vi "Main Tclk.vi"() -> ()   [LabVIEW 2018] (continued)
            n4776 = event-data() -> ()  [unwired: 5 out]
            n4777 = local read "SEM Scan Parameters"() -> (w3782:T26)
            n4778 = Unbundle By Name(w3782) -> ("X stig"=w3784:sgl[][], "X tiles"=w3780:u8, "Y tiles"=w3779:u8)
            n4779 = call "2D array edit.vi"("Data Entry Limits:Increment"=0.1, "Display Format:Precision"=u8 2, "Rows"=w3779, "Columns"=w3780, "Caption.Text"="X stig (%)", "Input array"=w3784) -> ("Output array"=w3777:sgl[][])  [unwired: 5 in]
            n4780 = Array Size(array=w3777) -> (size(s)=w3778:i32[])
            n4781 = Index Array(array=w3778) -> (element #1=w3776:i32, element #2=w3775:i32)  [unwired: 2 in]
            n4782 = Bundle By Name(cluster=w3782, "X stig"=w3777, "X tiles"=w3775, "Y tiles"=w3776) -> (w3781:T26)
            n4783 = local write "SEM Scan Parameters"(w3781) -> ()
          }
          event "SEM Scan Parameters.Y stig": Mouse Down; "SEM Scan Parameters.Y stig": Value Change {
            n4784 = event-data() -> ()  [unwired: 5 out]
            n4785 = local read "SEM Scan Parameters"() -> (w3794:T26)
            n4786 = Unbundle By Name(w3794) -> ("Y stig"=w3796:sgl[][], "X tiles"=w3792:u8, "Y tiles"=w3791:u8)
            n4787 = call "2D array edit.vi"("Data Entry Limits:Increment"=0.1, "Display Format:Precision"=u8 2, "Rows"=w3791, "Columns"=w3792, "Caption.Text"="Y stig (%)", "Input array"=w3796) -> ("Output array"=w3789:sgl[][])  [unwired: 5 in]
            n4788 = Array Size(array=w3789) -> (size(s)=w3790:i32[])
            n4789 = Index Array(array=w3790) -> (element #1=w3788:i32, element #2=w3787:i32)  [unwired: 2 in]
            n4790 = Bundle By Name(cluster=w3794, "Y stig"=w3789, "X tiles"=w3787, "Y tiles"=w3788) -> (w3793:T26)
            n4791 = local write "SEM Scan Parameters"(w3793) -> ()
          }
          event "SEM Scan Parameters.X aln": Mouse Down; "SEM Scan Parameters.X aln": Value Change {
            n4792 = event-data() -> ()  [unwired: 5 out]
            n4793 = local read "SEM Scan Parameters"() -> (w3806:T26)
            n4794 = Unbundle By Name(w3806) -> ("X aln"=w3808:sgl[][], "X tiles"=w3804:u8, "Y tiles"=w3803:u8)
            n4795 = call "2D array edit.vi"("Data Entry Limits:Increment"=0.1, "Display Format:Precision"=u8 2, "Rows"=w3803, "Columns"=w3804, "Caption.Text"="X aln (%)", "Input array"=w3808) -> ("Output array"=w3801:sgl[][])  [unwired: 5 in]
            n4796 = Array Size(array=w3801) -> (size(s)=w3802:i32[])
            n4797 = Index Array(array=w3802) -> (element #1=w3800:i32, element #2=w3799:i32)  [unwired: 2 in]
            n4798 = Bundle By Name(cluster=w3806, "X aln"=w3801, "X tiles"=w3799, "Y tiles"=w3800) -> (w3805:T26)
            n4799 = local write "SEM Scan Parameters"(w3805) -> ()
          }
          event "SEM Scan Parameters.Y aln": Mouse Down; "SEM Scan Parameters.Y aln": Value Change {
            n4800 = event-data() -> ()  [unwired: 5 out]
            n4801 = local read "SEM Scan Parameters"() -> (w3818:T26)
            n4802 = Unbundle By Name(w3818) -> ("Y aln"=w3820:sgl[][], "X tiles"=w3816:u8, "Y tiles"=w3815:u8)
            n4803 = call "2D array edit.vi"("Data Entry Limits:Increment"=0.1, "Display Format:Precision"=u8 2, "Rows"=w3815, "Columns"=w3816, "Caption.Text"="Y aln (%)", "Input array"=w3820) -> ("Output array"=w3813:sgl[][])  [unwired: 5 in]
            n4804 = Array Size(array=w3813) -> (size(s)=w3814:i32[])
            n4805 = Index Array(array=w3814) -> (element #1=w3811:i32, element #2=w3812:i32)  [unwired: 2 in]
            n4806 = Bundle By Name(cluster=w3818, "Y aln"=w3813, "X tiles"=w3812, "Y tiles"=w3811) -> (w3817:T26)
            n4807 = local write "SEM Scan Parameters"(w3817) -> ()
          }
          event "SEM Scan Parameters.dX (um)": Mouse Down {
            w3823 = u8 1 ("Rows")
            n4808 = event-data() -> ()  [unwired: 9 out]
            n4809 = local read "SEM Scan Parameters"() -> (w3831:T26)
            n4810 = local write "Delta X array for stop limit"(sgl[] [] ("Delta X array for stop limit")) -> ()
            n4811 = Unbundle By Name(w3831) -> ("dX (um)"=w3827:sgl[], "Y tiles"=w3822:u8)
            n4812 = Reshape Array(w3827, w3822, w3823) -> (w3826:sgl[][])
            n4813 = call "2D array edit.vi"("Data Entry Limits:Increment"=0.1, "Display Format:Precision"=u8 2, "Rows"=w3822, "Columns"=w3823, "Caption.Text"="dX (um)", "Input array"=w3826) -> ("Output array"=w3825:sgl[][])  [unwired: 5 in]
            n4814 = Reshape Array(w3825, w3822) -> (w3824:sgl[])
            n4815 = Bundle By Name(cluster=w3831, "dX (um)"=w3824, "Y tiles"=w3822) -> (w3830:T26)
            n4816 = local write "SEM Scan Parameters"(w3830) -> ()
          }
          event "SEM Scan Parameters.dY (um)": Mouse Down {
            w3838 = u8 1 ("Rows")
            n4817 = event-data() -> ()  [unwired: 9 out]
            n4818 = local read "SEM Scan Parameters"() -> (w3843:T26)
            n4819 = local write "Delta Y array for stop limit"(sgl[] [] ("Delta X array for stop limit")) -> ()
            n4820 = Unbundle By Name(w3843) -> ("dY (um)"=w3839:sgl[], "X tiles"=w3834:u8)
            n4821 = Reshape Array(w3839, w3838, w3834) -> (w3837:sgl[][])
            n4822 = call "2D array edit.vi"("Data Entry Limits:Increment"=0.1, "Display Format:Precision"=u8 2, "Rows"=w3838, "Columns"=w3834, "Caption.Text"="dY (um)", "Input array"=w3837) -> ("Output array"=w3836:sgl[][])  [unwired: 5 in]
            n4823 = Reshape Array(w3836, w3834) -> (w3835:sgl[])
            n4824 = Bundle By Name(cluster=w3843, "dY (um)"=w3835, "X tiles"=w3834) -> (w3842:T26)
            n4825 = local write "SEM Scan Parameters"(w3842) -> ()
          }
          event "X shift (nm/image)": Mouse Down {
            n4826 = event-data() -> ()  [unwired: 9 out]
            n4827 = local read "X shift (nm/image)"() -> (w3848:sgl)
            n4828 = local read "Remaining X shift frames"() -> (w3845:u32)
            n4829 = Compound Arithmetic op=MULTIPLY(w3848, sgl 0.001 ("value"), w3845) -> (w3849:sgl)
            n4830 = call "Image shift dialog.vi"("Remaining shift (um)"=w3849, "Image shift"=w3848, "Caption.Text"="X shift (nm/image)") -> ("Image shift (nm/image)"=w3850:sgl, "Remaining shift frames"=w3847:u32)  [unwired: 7 in]
            n4831 = local write "Remaining X shift frames"(w3847) -> ()
            n4832 = local write "X shift (nm/image)"(w3850) -> ()
          }
          event "Y shift (nm/image)": Mouse Down; "Y shift (nm/image)": Value Change {
            n4833 = event-data() -> ()  [unwired: 5 out]
            n4834 = local read "Y shift (nm/image)"() -> (w3855:sgl)
            n4835 = local read "Remaining Y shift frames"() -> (w3854:u32)
            n4836 = Compound Arithmetic op=MULTIPLY(w3855, sgl 0.001 ("value"), w3854) -> (w3856:sgl)
            n4837 = call "Image shift dialog.vi"("Remaining shift (um)"=w3856, "Image shift"=w3855, "Caption.Text"="Y shift (nm/image)") -> ("Image shift (nm/image)"=w3858:sgl, "Remaining shift frames"=w3853:u32)  [unwired: 7 in]
            n4838 = local write "Remaining Y shift frames"(w3853) -> ()
            n4839 = local write "Y shift (nm/image)"(w3858) -> ()
          }
          event "Mill": Value Change {
            n4840 = event-data() -> ("NewVal"=w3859:bool)  [unwired: 6 out]
            n4841 = case shown="True" w3859 {
              frame False {
                n4842 = local read "Original WatchDog Mode"() -> (w3860:u16)
                n4843 = shared-variable "My Computer\\Zeiss Library.lvlib\\Milling Stop"(TRUE ("Milling Stop")) -> ()  [unwired: 1 in, 1 out]
                n4844 = local write "WatchDog Mode"(w3860) -> ()
              }
              frame True {
                n4845 = stacked-sequence {
                  frame #0 {
                    n4846 = local read "WatchDog Mode"() -> (→"Original WatchDog Mode":u16)
                  }
                  frame #1 {
                    w3863 = u16 0 items=["Do Nothing", "Send Idle Only", "Watch FIB & SEM", "Watch FIB Only", "Watch SEM Only"] ("WatchDog Mode")
                    n4847 = local write "WatchDog Mode"(w3863) -> ()
                  }
                }
              }
            }
          }
          event "Mill Manual Pause": Value Change {
            w3869 = u8 0 ("AF Count")
            w3871 = FALSE ("Reset WD")
            w3870 = TRUE ("Reset WD")
            n4848 = event-data() -> ("NewVal"=w3872:bool)  [unwired: 5 out]
            n4849 = case shown="False" w3872 {
              frame False {
                n4850 = local read "Status message"() -> (w3883:string)
                n4851 = local read "Last milling snapshot"() -> (w3876:path)
                n4852 = Equal?(x=w3883, y="Manual pausing ..." ("Status message")) -> (x = y?=w3882:bool)
                n4853 = call-poly <vilib>:"Read From XML File.vi"("XML File Path"=w3876) -> ("XML Elements"=w3875:string)  [unwired: 8 in, 2 out]
                n4854 = Unflatten From XML(xml string=w3875, type=T46 {"Timestamp"=timestamp(0 s since 1904-01-01), "Milling Z voltage"=0.0, "FIB slice #"=0, "Pause for reheat"=FALSE, "Last good FI"=0.0, "Focus index"=0.0, "SEM max FOV"=0.0, "Remaining X shift frames"=0, "Remaining Y shift frames"=0} ("output cluster")) -> (value=w3877:T46)  [unwired: 1 in, 1 out]
                n4855 = Select(t="SEM between FIB" ("Status message"), s=w3882, f="Resume FIB milling ..." ("Status message")) -> (s? t:f=w3881:string)
                n4856 = Unbundle By Name(w3877) -> ("Milling Z voltage"=w3873:sgl)
                n4857 = shared-variable ".\\Zeiss Library.lvlib\\Milling Z Voltage Last"(w3873) -> ()  [unwired: 1 in, 1 out]
                n4858 = local write "Status message"(w3881) -> ()
              }
              frame True {
                n4859 = local read "Status message"() -> (w3889:string)
                n4860 = Equal?(x=w3889, y="SEM between FIB" ("Status message")) -> (x = y?=w3886:bool)
                n4861 = Select(t="Manual pausing ..." ("Status message"), s=w3886, f="Manual paused" ("Status message")) -> (s? t:f=w3885:string)
                n4862 = local write "Status message"(w3885) -> ()
              }
            }
            n4863 = local write "SW error warning armed"(w3870) -> ()
            n4864 = local write "Auto Focus"(w3871) -> ()
            n4865 = local write "Auto Stig"(w3871) -> ()
            n4866 = local write "Auto Align"(w3871) -> ()
            n4867 = local write "Reset Focus"(w3870) -> ()
            n4868 = local write "3D image paused armed"(w3870) -> ()
            n4869 = local write "Temperature warning armed"(w3870) -> ()
            n4870 = local write "AF Count"(w3869) -> ()
            n4871 = local write "AS Count"(w3869) -> ()
            n4872 = local write "AA Count"(w3869) -> ()
            n4873 = local read "SEM Scan Parameters"() -> (w3865:T26)
            n4874 = Unbundle By Name(w3865) -> ("Y tiles"=w3866:u8, "X tiles"=w3867:u8)
            n4875 = Initialize Array(FALSE ("ASX Success"), w3866, w3867) -> (w3868:bool[][])
            n4876 = local write "AAY Success tiled"(w3868) -> ()
            n4877 = local write "AF Success tiled"(w3868) -> ()
            n4878 = local write "ASX Success tiled"(w3868) -> ()
            n4879 = local write "ASY Success tiled"(w3868) -> ()
            n4880 = local write "AAX Success tiled"(w3868) -> ()
          }
          event "Mill Stop": Value Change {
            n4881 = event-data() -> ("NewVal"=w3890:bool)  [unwired: 6 out]
            n4882 = case shown="True" w3890 {
              frame False {
              }
              frame True {
                n4883 = local read "Original WatchDog Mode"() -> (w3891:u16)
                n4884 = shared-variable "My Computer\\Zeiss Library.lvlib\\Milling Stop"(TRUE ("Milling Stop")) -> ()  [unwired: 1 in, 1 out]
                n4885 = local write "WatchDog Mode"(w3891) -> ()
              }
            }
          }
          event "Save Probe Table": Value Change {
            n4886 = event-data() -> ("NewVal"=w3893:bool)  [unwired: 5 out]
            n4887 = case shown="True" w3893 {
              frame False {
              }
              frame True {
                n4888 = Two Button Dialog(message="Save FIB Probe Table?") -> (T button?=w3894:bool)  [unwired: 2 in]
                n4889 = case shown="True" w3894 {
                  frame False {
                    n4890 = local write "Save Probe Table"(FALSE ("Min FIB probe")) -> ()
                  }
                  frame True {
                    n4891 = stacked-sequence {
                      frame #0 {
                        n4892 = local read "Api"() -> (w3898:refnum<k7>)
                        n4893 = local read "FIB Milling Probe"() -> (w3897:string)
                        n4894 = call "SmartSEM Remote API save FIB probe table.vi"("FIB Probe"=w3897, "ActiveX Container"=w3898) -> ()  [unwired: 8 in, 2 out]
                        n4895 = local write "Status message"("Measuring FIB probe currents" ("Status message")) -> ()
                      }
                      frame #1 {
                        n4896 = local write "Save Probe Table"(FALSE ("Min FIB probe")) -> ()
                        n4897 = local write "Status message"("FIB Probe Table saved" ("Status message")) -> ()
                      }
                    }
                  }
                }
              }
            }
          }
          event "FIB Milling Probe": Value Change {
            n4898 = event-data() -> ()  [unwired: 6 out]
            n4899 = local read "Machine Type"() -> (w3902:u8)
            n4900 = case shown="2" w3902 {
              frame 0, Default {
              }
              frame 2 {
                n4901 = local read "Api"() -> (w3909:refnum<k7>)
                n4902 = call "SmartSEM Remote API set string.vi"("vValue"="FIB Milling Probe", "lpszParam"="DP_FIB_IMAGE_PROBE", "ActiveX Container"=w3909) -> ("error out"=w3903:errorcluster, "reference out"=w3906:refnum<k7>)  [unwired: 7 in]
                n4903 = call "SmartSEM Remote API set string.vi"("error in"=w3903, "vValue"="Undefined", "lpszParam"="DP_FIB_MILL_PROBE", "ActiveX Container"=w3906) -> ()  [unwired: 6 in, 2 out]
              }
            }
          }
          event "Min FIB probe": Value Change {
            n4904 = event-data() -> ("NewVal"=w3910:bool)  [unwired: 5 out]
            n4905 = case shown="True" w3910 {
              frame False {
              }
              frame True {
                n4906 = Two Button Dialog(message="Switch to min current of the same probe size?") -> (T button?=w3911:bool)  [unwired: 2 in]
                n4907 = case shown="True" w3911 {
                  frame False {
                    n4908 = local write "Min FIB probe"(FALSE ("Min FIB probe")) -> ()
                  }
                  frame True {
                    n4909 = stacked-sequence {
                      frame #0 {
                        n4910 = local read "Api"() -> (w3916:refnum<k7>)
                        n4911 = local read "FIB Milling Probe"() -> (w3917:string)
                        n4912 = local write "Min FIB probe"(FALSE ("Min FIB probe")) -> ()
                        n4913 = call "SmartSEM Remote API goto min or max FIB probe current.vi"("Min or Max"="Min", "FIB Probe"=w3917, "ActiveX Container"=w3916) -> ("Goto probe"=w3914:string)  [unwired: 7 in, 1 out]
                        n4914 = local write "FIB Milling Probe"(w3914) -> ()
                        n4915 = local write "Status message"("Measuring FIB probe currents" ("Status message")) -> ()
                      }
                      frame #1 {
                        n4916 = local write "Status message"("Switched to minimal current of the same probe" ("Status message")) -> ()
                      }
                    }
                  }
                }
              }
            }
          }
          event "Max FIB probe": Value Change {
            n4917 = event-data() -> ("NewVal"=w3921:bool)  [unwired: 5 out]
            n4918 = case shown="True" w3921 {
              frame False {
              }
              frame True {
                n4919 = Two Button Dialog(message="Switch to max current of the same probe size?") -> (T button?=w3922:bool)  [unwired: 2 in]
                n4920 = case shown="True" w3922 {
                  frame False {
                    n4921 = local write "Max FIB probe"(FALSE ("Min FIB probe")) -> ()
                  }
                  frame True {
                    n4922 = stacked-sequence {
                      frame #0 {
                        n4923 = local read "Api"() -> (w3928:refnum<k7>)
                        n4924 = local read "FIB Milling Probe"() -> (w3927:string)
                        n4925 = local write "Max FIB probe"(FALSE ("Min FIB probe")) -> ()
                        n4926 = call "SmartSEM Remote API goto min or max FIB probe current.vi"("Min or Max"="Max", "FIB Probe"=w3927, "ActiveX Container"=w3928) -> ("Goto probe"=w3926:string)  [unwired: 7 in, 1 out]
                        n4927 = local write "FIB Milling Probe"(w3926) -> ()
                        n4928 = local write "Status message"("Measuring FIB probe currents" ("Status message")) -> ()
                      }
                      frame #1 {
                        n4929 = local write "Status message"("Switched to maximal current of the same probe" ("Status message")) -> ()
                      }
                    }
                  }
                }
              }
            }
          }
          event "FIB time lapse": Value Change {
            n4930 = event-data() -> ("NewVal"=w3932:bool)  [unwired: 5 out]
            n4931 = case shown="False" w3932 {
              frame False {
                n4932 = stacked-sequence {
                  frame #0 {
                    n4933 = local read "FIB HW Config"() -> (w3935:T23)
                    n4934 = Unbundle By Name(w3935) -> ("Beam blank"=w3936:tag)
                    n4935 = local read "Api"() -> (w3933:refnum<k7>)
                    n4936 = call "FIB beam blank.vi"("ActiveX Container"=w3933, "Beam blanked"=TRUE ("Ext on"), "lines"=w3936) -> ()  [unwired: 2 in, 1 out]
                  }
                  frame #1 {
                    n4937 = local read "SEM HW Config"() -> (w3941:T9)
                    n4938 = Unbundle By Name(w3941) -> ("Detector FIB-NI auto switch"=w3942:tag)
                    n4939 = call-poly <vilib>:"DAQmx Create Virtual Channel.vi"("lines"=w3942) -> ("task out"=w3939:refnum<k21>, "error out"=w3940:errorcluster)  [unwired: 4 in, 9 out]
                    n4940 = call-poly <vilib>:"DAQmx Write.vi"("task/channels in"=w3939, "data"=FALSE, "error in"=w3940) -> ("task out"=w3937:refnum<k21>, "error out"=w3938:errorcluster)  [unwired: 1 in, 10 out]
                    n4941 = call <vilib>:"DAQmx Clear Task.vi"("task in"=w3937, "error in"=w3938) -> ()  [unwired: 14 out]
                  }
                  frame #2 {
                    n4942 = local read "FIB HW Config"() -> (w3946:T23)
                    n4943 = Unbundle By Name(w3946) -> ("FIB Ext Scan"=w3945:tag)
                    n4944 = call "FIB ext scan.vi"("Ext on"=FALSE, "FIB Ext Scan"=w3945) -> ()  [unwired: 9 in, 1 out]
                  }
                  frame #3 {
                    n4945 = local read "Machine Type"() -> (w3947:u8)
                    n4946 = case shown="2" w3947 {
                      frame 0, Default {
                      }
                      frame 1 {
                        w3948 = TRUE ("Initialization")
                        n4947 = local read "COM port"() -> (w3954:refnum<visa-resource-name>)
                        n4948 = call "FIB mode.vi"("Initialization"=w3948, "FIB mode"=T10."SEM", "COM port in"=w3954) -> ("COM port out"=w3953:refnum<visa-resource-name>)  [unwired: 7 in, 1 out]
                        n4949 = call "Remcon32 command.vi"("SEM command"="edx 0", "COM port in"=w3953) -> ("COM port out"=w3952:refnum<visa-resource-name>)  [unwired: 6 in, 3 out]
                        n4950 = call "Remcon32 command.vi"("Close session"=w3948, "SEM command"="frez", "COM port in"=w3952) -> ()  [unwired: 5 in, 4 out]
                      }
                      frame 2 {
                        n4951 = local read "Api"() -> (w3955:refnum<k7>)
                        n4952 = call "SmartSEM Remote API set float.vi"("vValue"=sgl 2.0, "lpszParam"="DP_FIB_BLANKER_MODE" ("lpszCommand"), "ActiveX Container"=w3955) -> ("error out"=w3956:errorcluster, "reference out"=w3957:refnum<k7>)  [unwired: 7 in]
                        n4953 = call "SmartSEM Remote API FIB mode.vi"("error in"=w3956, "FIB mode"=T50."SEM", "ActiveX Container"=w3957) -> ("error out"=w3960:errorcluster, "reference out"=w3961:refnum<k7>)  [unwired: 7 in]
                        n4954 = invoke class="_EMApi" method="Execute"(reference=w3961, error in=w3960, "lpszCommand"="CMD_FREEZE_ALL") -> ()  [unwired: 1 in, 4 out]
                      }
                    }
                  }
                  frame #4 {
                    n4955 = local write "Status message"("standby" ("Status message")) -> ()
                  }
                }
              }
              frame True {
              }
            }
          }
          event "FIB Image": Mouse Down {
            n4956 = event-data() -> ("Coords"=→"Mouse Down Coords":T22)  [unwired: 3 out]
            n4957 = register-events(reference=w3973, w3969) -> (reference out=w3972:refnum<event-registration>, error out=w3971:errorcluster)  [unwired: 1 in]
            n4958 = local read "Spot"() -> (w3968:bool)
            n4959 = property on="Cursor Z (V)" class="DigNum (strict)"("Visible"=FALSE) -> ()  [unwired: 2 in, 2 out]
            n4960 = case shown="False" w3968 {
              frame False {
              }
              frame True {
                n4961 = local read "FIB HW Config"() -> (w3977:T23)
                n4962 = Unbundle By Name(w3977) -> ("Beam blank"=w3976:tag)
                n4963 = local read "Api"() -> (w3974:refnum<k7>)
                n4964 = call "FIB beam blank.vi"("ActiveX Container"=w3974, "Beam blanked"=TRUE, "lines"=w3976) -> ()  [unwired: 2 in, 1 out]
              }
            }
            "Mouse down" <- TRUE ("Mouse down")
          }
          event "FIB Image": Mouse Move {
            n4965 = event-data() -> ("Coords"=w3982:T22)  [unwired: 1 out]
            n4966 = local read "Mouse down"() -> (w3981:bool)
            n4967 = local read "Spot"() -> (w3980:bool)
            n4968 = local read "FIB"() -> (w3979:bool)
            n4969 = Or(x=w3980, y=w3979) -> (x .or. y?=w3978:bool)
            n4970 = case shown="False" w3981 {
              tunnel: [w4009 w4013] -> w3984
              tunnel: w3983 -> [w4009 w4012]
              tunnel: w3982 -> [w4008 w4011]
              tunnel: w3978 -> [_ w4010]
              frame False {
                w3985 = i16 0 ("upper limit")
                n4971 = property on="FIB Image" class="IntGraph (strict)"() -> ("Plot Bounds"=w4007:T70, "Width"=w3989:u32, "Height"=w3997:u32)  [unwired: 2 in, 2 out]
                n4972 = local read "FIB Scan Parameters"() -> (w4006:T32)
                n4973 = Unbundle By Name(w4007) -> ("Right"=w3992:i16, "Bottom"=w4000:i16)
                n4974 = Unbundle By Name(w4008) -> ("Horizontal"=w3991:i32, "Vertical"=w3993:i32)
                n4975 = Unbundle By Name(w4006) -> ("Z size (V)"=w3999:dbl)
                n4976 = To Word Integer(number=w3997) -> (16bit integer=w3995:i16)
                n4977 = To Word Integer(number=w3993) -> (16bit integer=w3994:i16)
                n4978 = Subtract(x=w3992, y=w3991) -> (x-y=w3990:i32)
                n4979 = Subtract(x=w4000, y=w3994) -> (x-y=w3996:i16)
                n4980 = In Range and Coerce(upper limit=w3989, x=w3990, lower limit=w3985) -> (In Range?=w3988:bool)  [unwired: 1 out]
                n4981 = In Range and Coerce(upper limit=w3995, x=w3996, lower limit=w3985) -> (coerced(x)=w3998:i16, In Range?=w3987:bool)
                n4982 = Multiply(x=w3998, y=w3999) -> (x*y=w4005:dbl)
                n4983 = Multiply(x=w3999, y=0.5) -> (x*y=w4003:dbl)
                n4984 = And(x=w3988, y=w3987) -> (x .and. y?=w3986:bool)
                n4985 = Divide(x=w4005, y=w3997) -> (x/y=w4004:dbl)
                n4986 = property on="Cursor Z (V)" class="DigNum (strict)"("Visible"=w3986) -> ()  [unwired: 2 in, 2 out]
                n4987 = Subtract(x=w4004, y=w4003) -> (x-y=→"Cursor Z (V)":dbl)
              }
              frame True {
                n4988 = case shown="False" w4010 {
                  tunnel: w4011 -> [w4015 _]
                  tunnel: [w4014 w4138] -> w4013
                  tunnel: w4012 -> [_ w4138]
                  frame False {
                    n4989 = stacked-sequence {
                      tunnel: w4015 -> [_ w4020]
                      tunnel: [_ w4018] -> w4014
                      frame #0 {
                        n4990 = call <vilib>:"Draw Rectangle.vi"("picture"=picture data[5B]) -> ("new picture"=w4017:picture)  [unwired: 8 in]
                        n4991 = property on="FIB Image" class="IntGraph (strict)"("PlotImages.Front"=w4017) -> ()  [unwired: 2 in, 2 out]
                      }
                      frame #1 {
                        n4992 = case shown="True" "ROI" {
                          tunnel: w4020 -> [w4062 w4129]
                          tunnel: [w4021 w4073] -> w4018
                          frame False {
                            w4039 = 5 ("dimension size")
                            w4060 = u32 16711680 ("color(black)")
                            n4993 = local read "Mouse Down Coords"() -> (w4063:T22)
                            n4994 = Subtract(x=w4062, y=w4063) -> (x-y=w4061:T22)
                            n4995 = Unbundle By Name(w4061) -> ("Horizontal"=w4040:i32, "Vertical"=w4038:i32)
                            n4996 = Initialize Array(w4040, w4039) -> (w4037:i32[])
                            n4997 = Initialize Array(w4038, w4039) -> (w4036:i32[])
                            n4998 = local read "FIB Scan Parameters"() -> (w4050:T32)
                            n4999 = local read "Milling para"() -> (w4055:T35)
                            n5000 = local read "FIB Options"() -> (w4056:T33)
                            n5001 = local read "Trapezoidal"() -> (w4022:cluster{"X":i16, "Y":i16}[])
                            n5002 = Build Cluster Array(w4037, w4036) -> (w4035:cluster{"Horizontal":i32, "Vertical":i32}[])
                            n5003 = To Word Integer(number=w4035) -> (16bit integer=w4034:cluster{"Horizontal":i16, "Vertical":i16}[])
                            n5004 = Unbundle By Name(w4055) -> ("Mill from Bottom"=w4054:bool)
                            n5005 = Unbundle By Name(w4056) -> ("Flip z"=w4042:bool)
                            n5006 = Add(x=w4034, y=w4022) -> (x+y=w4021:cluster{i16, i16}[])
                            n5007 = Unbundle By Name(w4050) -> ("Z size (V)"=w4051:dbl)
                            n5008 = for {
                              tunnel: w4021 -> [w4072] mode=indexing
                              tunnel: [w4071] -> w4033 mode=indexing
                              tunnel: [w4070] -> w4028 mode=indexing
                              n5009 = Unbundle(w4072) -> (w4071:i16, w4070:i16)
                            }
                            n5010 = Exclusive Or(1:w4042, 2:w4054) -> (0:w4025:bool)
                            n5011 = case shown="False" w4025 {
                              tunnel: [2 ("index") 0 ("index")] -> w4032
                              tunnel: [3 ("index") 1 ("index")] -> w4031
                              frame False {
                              }
                              frame True {
                              }
                            }
                            n5012 = Index Array(array=w4028, index #1=0 ("index"), index #2=2 ("index")) -> (element #1=w4027:i16, element #2=w4026:i16)
                            n5013 = Index Array(array=w4033, index #1=w4032, index #2=w4031) -> (element #1=w4023:i16, element #2=w4024:i16)
                            n5014 = Select(t=w4027, s=w4025, f=w4026) -> (s? t:f=w4041:i16)
                            n5015 = property on="FIB Image" class="IntGraph (strict)"() -> ("Height"=w4049:u32)  [unwired: 2 in, 2 out]
                            n5016 = Divide(x=w4041, y=w4049) -> (x/y=w4048:dbl)
                            n5017 = Subtract(x=w4048, y=0.5) -> (x-y=w4046:dbl)
                            n5018 = call <vilib>:"Draw Multiple Lines.vi"("picture"=picture data[5B], "line endpoints"=w4021, "color(black)"=u32 6618880) -> ("new picture"=w4059:picture)  [unwired: 6 in]
                            n5019 = Multiply(x=w4046, y=w4051) -> (x*y=w4045:dbl)
                            n5020 = Bundle(w4023, w4041) -> (w4053:cluster{i16, i16})  [unwired: 1 in]
                            n5021 = Bundle(w4024, w4041) -> (w4052:cluster{i16, i16})  [unwired: 1 in]
                            n5022 = Negate(x=w4045) -> (-x=w4044:dbl)
                            n5023 = call <vilib>:"Draw Point.vi"("picture"=w4059, "point(x,y)"=w4053, "color(black)"=w4060) -> ("new picture"=w4058:picture)  [unwired: 6 in]
                            n5024 = Select(t=w4044, s=w4042, f=w4045) -> (s? t:f=w4043:dbl)
                            n5025 = call <vilib>:"Draw Line.vi"("picture"=w4058, "end point"=w4052, "color(black)"=w4060) -> ("new picture"=w4057:picture)  [unwired: 6 in]
                            n5026 = shared-variable ".\\Zeiss Library.lvlib\\Milling Z Voltage RT"(w4043) -> ()  [unwired: 1 in, 1 out]
                            n5027 = property on="FIB Image" class="IntGraph (strict)"("PlotImages.Front"=w4057) -> ()  [unwired: 2 in, 2 out]
                          }
                          frame True {
                            w4109 = u32 16711680 ("color(black)")
                            w4113 = T47 {"left"=0, "top"=0, "right"=0, "bottom"=0} ("rect")
                            n5028 = local read "Mouse Down Coords"() -> (w4128:T22)
                            n5029 = property on="FIB Image" class="IntGraph (strict)"() -> ("Plot Bounds"=w4112:T70)  [unwired: 2 in, 2 out]
                            n5030 = Unbundle By Name(w4129) -> ("Horizontal"=w4127:i32, "Vertical"=w4125:i32)
                            n5031 = Unbundle By Name(w4128) -> ("Horizontal"=w4126:i32, "Vertical"=w4124:i32)
                            n5032 = local read "FIB Scan Parameters"() -> (w4102:T32)
                            n5033 = local read "Milling para"() -> (w4096:T35)
                            n5034 = local read "FIB Options"() -> (w4106:T33)
                            n5035 = Unbundle By Name(w4112) -> ("Left"=w4119:i16, "Top"=w4118:i16)
                            n5036 = Unbundle By Name(w4112) -> ("Left"=w4117:i16, "Top"=w4116:i16)
                            n5037 = Max & Min(x=w4127, y=w4126) -> (max(x,y)=w4123:i32, min(x,y)=w4122:i32)
                            n5038 = Max & Min(x=w4125, y=w4124) -> (max(x,y)=w4120:i32, min(x,y)=w4121:i32)
                            n5039 = Bundle By Name(cluster=w4113, "left"=w4122, "top"=w4121, "right"=w4123, "bottom"=w4120) -> (w4115:T47)
                            n5040 = Bundle By Name(cluster=w4113, "left"=w4119, "top"=w4118, "right"=w4117, "bottom"=w4116) -> (w4114:T47)
                            n5041 = Unbundle By Name(w4096) -> ("Mill from Bottom"=w4094:bool)
                            n5042 = Unbundle By Name(w4106) -> ("Flip z"=w4093:bool)
                            n5043 = Unbundle By Name(w4102) -> ("Z size (V)"=w4100:dbl)
                            n5044 = Subtract(x=w4115, y=w4114) -> (x-y=w4075:T47)
                            n5045 = Unbundle By Name(w4075) -> ("left"=w4091:i16, "top"=w4081:i16, "right"=w4088:i16, "bottom"=w4080:i16)
                            n5046 = Exclusive Or(1:w4093, 2:w4094) -> (0:w4092:bool)
                            n5047 = Select(t=w4081, s=w4092, f=w4080) -> (s? t:f=w4095:i16)
                            n5048 = property on="FIB Image" class="IntGraph (strict)"() -> ("Height"=w4105:u32)  [unwired: 2 in, 2 out]
                            n5049 = Initialize Array(w4091, 5 ("dimension size")) -> (w4089:i16[])
                            n5050 = Initialize Array(w4081, 5 ("dimension size")) -> (w4082:i16[])
                            n5051 = Divide(x=w4095, y=w4105) -> (x/y=w4104:dbl)
                            n5052 = Subtract(x=w4104, y=0.5) -> (x-y=w4101:dbl)
                            n5053 = Replace Array Subset(array=w4089, new element #1=w4088, index #1=1 ("index"), new element #2=w4088, index #2=2 ("index")) -> (w4079:i16[])
                            n5054 = Replace Array Subset(array=w4082, new element #1=w4080, index #1=2 ("index"), new element #2=w4080, index #2=3 ("index")) -> (w4078:i16[])
                            n5055 = Multiply(x=w4101, y=w4100) -> (x*y=w4099:dbl)
                            n5056 = Build Cluster Array(w4079, w4078) -> (w4073:cluster{"left":i16, "top":i16}[])
                            "Trapezoidal" <- w4073
                            n5057 = Negate(x=w4099) -> (-x=w4098:dbl)
                            n5058 = Select(t=w4098, s=w4093, f=w4099) -> (s? t:f=w4097:dbl)
                            n5059 = shared-variable ".\\Zeiss Library.lvlib\\Milling Z Voltage RT"(w4097) -> ()  [unwired: 1 in, 1 out]
                            n5060 = call <vilib>:"Draw Multiple Lines.vi"("picture"=picture data[5B], "line endpoints"=w4073, "color(black)"=u32 6618880) -> ("new picture"=w4074:picture)  [unwired: 6 in]
                            n5061 = Bundle("left"=w4091, "bottom"=w4095) -> (w4110:cluster{"left":i16, "bottom":i16})  [unwired: 1 in]
                            n5062 = Bundle("right"=w4088, "bottom"=w4095) -> (w4108:cluster{"right":i16, "bottom":i16})  [unwired: 1 in]
                            n5063 = call <vilib>:"Draw Point.vi"("picture"=w4074, "point(x,y)"=w4110, "color(black)"=w4109) -> ("new picture"=w4111:picture)  [unwired: 6 in]
                            n5064 = call <vilib>:"Draw Line.vi"("picture"=w4111, "end point"=w4108, "color(black)"=w4109) -> ("new picture"=w4107:picture)  [unwired: 6 in]
                            n5065 = property on="FIB Image" class="IntGraph (strict)"("PlotImages.Front"=w4107) -> ()  [unwired: 2 in, 2 out]
                          }
                        }
                      }
                    }
                  }
                  frame True {
                    w4134 = 1.0 ("upper limit")
                    w4135 = 511.0 ("upper limit")
                    w4136 = 0.0 ("Y Scale.Range:Minimum")
                    w4137 = 512.0 ("X Scale.Range:Maximum")
                    n5066 = property on="FIB Image" class="IntGraph (strict)"("XScale.Maximum"=w4137, "XScale.Minimum"=w4136, "YScale.Maximum"=w4137, "YScale.Minimum"=w4136) -> ("Cursor.Cursor X"=w4133:dbl, "Cursor.Cursor Y"=w4132:dbl)  [unwired: 2 in, 2 out]
                    n5067 = In Range and Coerce(upper limit=w4135, x=w4133, lower limit=w4134) -> (coerced(x)=w4131:dbl)  [unwired: 1 out]
                    n5068 = In Range and Coerce(upper limit=w4135, x=w4132, lower limit=w4134) -> (coerced(x)=w4130:dbl)  [unwired: 1 out]
                    n5069 = property on="FIB Image" class="IntGraph (strict)"("Cursor.Cursor X"=w4131, "Cursor.Cursor Y"=w4130) -> ()  [unwired: 2 in, 2 out]
                  }
                }
              }
            }
          }
          event "FIB Image": Mouse Up {
            w4143 = i16 0 ("upper limit")
            n5070 = event-data() -> ("Coords"=w4142:T22)  [unwired: 3 out]
            n5071 = local read "Mouse Down Coords"() -> (w4172:T22)
            n5072 = property on="FIB Image" class="IntGraph (strict)"() -> ("Plot Bounds"=w4164:T70, "Width"=w4147:u32, "Height"=w4155:u32)  [unwired: 2 in, 2 out]
            n5073 = local read "FIB Scan Parameters"() -> (w4163:T32)
            n5074 = Equal?(x=w4172, y=w4142) -> (x = y?=w4171:cluster{"Horizontal":bool, "Vertical":bool})
            n5075 = Unbundle By Name(w4164) -> ("Right"=w4150:i16, "Bottom"=w4158:i16)
            n5076 = Unbundle By Name(w4142) -> ("Horizontal"=w4149:i32, "Vertical"=w4151:i32)
            n5077 = Unbundle By Name(w4171) -> ("Horizontal"=w4169:bool, "Vertical"=w4170:bool)
            n5078 = register-events(reference=w4176, refnum<k0> refnum) -> (reference out=w4175:refnum<event-registration>, error out=w4174:errorcluster)  [unwired: 1 in]
            n5079 = local write "Mouse down"(FALSE ("Mouse down")) -> ()
            n5080 = local read "Spot"() -> (w4139:bool)
            n5081 = local read "FIB"() -> (w4168:bool)
            n5082 = Unbundle By Name(w4163) -> ("Z size (V)"=w4157:dbl)
            n5083 = To Word Integer(number=w4155) -> (16bit integer=w4153:i16)
            n5084 = To Word Integer(number=w4151) -> (16bit integer=w4152:i16)
            n5085 = Subtract(x=w4150, y=w4149) -> (x-y=w4148:i32)
            n5086 = Subtract(x=w4158, y=w4152) -> (x-y=w4154:i16)
            n5087 = And(x=w4169, y=w4170) -> (x .and. y?=w4167:bool)
            n5088 = In Range and Coerce(upper limit=w4147, x=w4148, lower limit=w4143) -> (In Range?=w4146:bool)  [unwired: 1 out]
            n5089 = In Range and Coerce(upper limit=w4153, x=w4154, lower limit=w4143) -> (coerced(x)=w4156:i16, In Range?=w4145:bool)
            n5090 = Compound Arithmetic op=OR(w4139, w4168, w4167) -> (w4166:bool)
            n5091 = Multiply(x=w4156, y=w4157) -> (x*y=w4162:dbl)
            n5092 = Multiply(x=w4157, y=0.5) -> (x*y=w4160:dbl)
            n5093 = And(x=w4146, y=w4145) -> (x .and. y?=w4144:bool)
            n5094 = Divide(x=w4162, y=w4155) -> (x/y=w4161:dbl)
            n5095 = property on="Cursor Z (V)" class="DigNum (strict)"("Visible"=w4144) -> ()  [unwired: 2 in, 2 out]
            n5096 = Subtract(x=w4161, y=w4160) -> (x-y=w4141:dbl)
            n5097 = local write "Cursor Z (V)"(w4141) -> ()
            n5098 = case shown="True" w4166 {
              tunnel: w4140 -> [w4182 _]
              tunnel: w4139 -> [_ w4249]
              frame False {
                n5099 = for {
                  tunnel: w4182 -> [w4240] mode=indexing
                  tunnel: [w4239] -> w4216 mode=indexing
                  tunnel: [w4238] -> w4193 mode=indexing
                  n5100 = Unbundle(w4240) -> ("X"=w4239:i16, "Y"=w4238:i16)
                }
                n5101 = local write "Trapezoidal"(w4182) -> ()
                n5102 = property on="FIB Image" class="IntGraph (strict)"() -> ("Height"=w4192:u32, "Width"=w4205:u32)  [unwired: 2 in, 2 out]
                n5103 = Divide(x=w4192, y=w4205) -> (x/y=w4233:dbl)
                n5104 = Index Array(array=w4216, index #1=1 ("index"), index #2=2 ("index"), index #3=0 ("index"), index #4=3 ("index")) -> (element #1=w4186:i16, element #2=w4187:i16, element #3=w4188:i16, element #4=w4213:i16)
                n5105 = Index Array(array=w4193, index #1=2 ("index"), index #2=3 ("index"), index #3=0 ("index"), index #4=1 ("index")) -> (element #1=w4183:i16, element #2=w4184:i16, element #3=w4185:i16, element #4=w4198:i16)
                n5106 = local read "Milling para"() -> (w4235:T35)
                n5107 = Add(x=w4186, y=w4187) -> (x+y=w4212:i16)
                n5108 = Add(x=w4188, y=w4213) -> (x+y=w4211:i16)
                n5109 = Add(x=w4183, y=w4184) -> (x+y=w4199:i16)
                n5110 = Add(x=w4185, y=w4198) -> (x+y=w4200:i16)
                n5111 = expression code="x*2"(w4205) -> (w4209:u32)
                n5112 = expression code="x*2"(w4192) -> (w4202:u32)
                n5113 = Unbundle By Name(w4235) -> ("FIB FOV (um)"=w4234:sgl, "Z-step (nm)"=w4177:dbl)
                n5114 = Add(x=w4212, y=w4211) -> (x+y=w4210:i16)
                n5115 = Subtract(x=w4212, y=w4211) -> (x-y=w4206:i16)
                n5116 = Add(x=w4199, y=w4200) -> (x+y=w4201:i16)
                n5117 = Subtract(x=w4199, y=w4200) -> (x-y=w4204:i16)
                n5118 = Divide(x=w4210, y=w4209) -> (x/y=w4208:dbl)
                n5119 = Divide(x=w4206, y=w4205) -> (x/y=w4190:dbl)
                n5120 = Divide(x=w4201, y=w4202) -> (x/y=w4203:dbl)
                n5121 = Divide(x=w4204, y=w4192) -> (x/y=w4189:dbl)
                n5122 = Decrement(x=w4208) -> (x-1=w4207:dbl)
                n5123 = Decrement(x=w4203) -> (x-1=w4191:dbl)
                n5124 = expression code="x/2"(w4234) -> (w4223:sgl)
                n5125 = expression code="x/1e3"(w4177) -> (w4222:dbl)
                n5126 = Compound Arithmetic op=MULTIPLY(w4189, w4223, w4233) -> (w4232:dbl)
                n5127 = Divide(x=w4232, y=w4222) -> (x/y=w4231:dbl)
                n5128 = Round To Nearest(number=w4231) -> (nearest integer value=w4219:dbl)
                n5129 = Multiply(x=w4207, y=w4223) -> (x*y=w4224:dbl)
                n5130 = Multiply(x=w4191, y=w4223) -> (x*y=w4225:dbl)
                n5131 = Multiply(x=w4190, y=w4223) -> (x*y=w4226:dbl)
                n5132 = Multiply(x=w4219, y=w4222) -> (x*y=w4221:dbl)
                n5133 = Round To Nearest(number=w4224) -> (nearest integer value=w4181:dbl)
                n5134 = Round To Nearest(number=w4225) -> (nearest integer value=w4180:dbl)
                n5135 = expression code="log2( x/0.1)"(w4226) -> (w4228:dbl)
                n5136 = Round To Nearest(number=w4226) -> (nearest integer value=w4179:dbl)
                n5137 = Round To Nearest(number=w4221) -> (nearest integer value=w4178:dbl)
                n5138 = Round Toward +Infinity(x=w4228) -> (ceil(x): smallest int >= x=w4230:dbl)
                n5139 = Increment(x=w4219) -> (x+1=w4220:dbl)
                n5140 = Scale By Power Of 2(n=w4230, x=ext 1.0) -> (x*2^n=w4227:ext)
                n5141 = local read "Milling para"() -> (w4236:T35)
                n5142 = Bundle By Name(cluster=w4236, "X center (um)"=w4181, "Z center (um)"=w4180, "X size (um)"=w4179, "Z size (um)"=w4178, "Z resolution"=w4220, "X resolution"=w4227) -> (w4237:T35)
                n5143 = local write "Milling para"(w4237) -> ()
              }
              frame True {
                w4243 = 1.0 ("upper limit")
                w4244 = 511.0 ("upper limit")
                w4247 = 0.0 ("Y Scale.Range:Minimum")
                w4248 = 512.0 ("X Scale.Range:Maximum")
                n5144 = case shown="True" w4249 {
                  frame False {
                  }
                  frame True {
                    n5145 = local read "FIB HW Config"() -> (w4253:T23)
                    n5146 = Unbundle By Name(w4253) -> ("Beam blank"=w4252:tag)
                    n5147 = local read "Api"() -> (w4250:refnum<k7>)
                    n5148 = call "FIB beam blank.vi"("ActiveX Container"=w4250, "Beam blanked"=FALSE, "lines"=w4252) -> ()  [unwired: 2 in, 1 out]
                  }
                }
                n5149 = property on="FIB Image" class="IntGraph (strict)"("XScale.Maximum"=w4248, "XScale.Minimum"=w4247, "YScale.Maximum"=w4248, "YScale.Minimum"=w4247) -> ("Cursor.Cursor X"=w4246:dbl, "Cursor.Cursor Y"=w4245:dbl)  [unwired: 2 in, 2 out]
                n5150 = In Range and Coerce(upper limit=w4244, x=w4246, lower limit=w4243) -> (coerced(x)=w4242:dbl)  [unwired: 1 out]
                n5151 = In Range and Coerce(upper limit=w4244, x=w4245, lower limit=w4243) -> (coerced(x)=w4241:dbl)  [unwired: 1 out]
                n5152 = property on="FIB Image" class="IntGraph (strict)"("Cursor.Cursor X"=w4242, "Cursor.Cursor Y"=w4241) -> ()  [unwired: 2 in, 2 out]
              }
            }
          }
          event "SEM Shutter": Value Change {
            # "Turn on the e-mail warning mechanism because of the failed attempt."
            n5153 = event-data() -> ("NewVal"=w4261:bool)  [unwired: 1 out]
            n5154 = local read "Hardware Configuration"() -> (w4260:T25)
            n5155 = Unbundle By Name(w4260) -> ("Shutter Drive"=w4259:tag)
            n5156 = local read "Damping"() -> (w4254:bool)
            n5157 = call "Shutter Swing V3.vi"("Shutter Drive"=w4259, "Damping"=w4254, "Shutter close"=w4261) -> ("Shutter close fdbk"=w4257:bool, "Fail #"=w4256:u8, "SEM shutter status"=→"SEM shutter status":string)  [unwired: 2 in, 4 out]
            "Fail #" <- w4256
            n5158 = Greater Than 0?(x=w4256) -> (x > 0?=w4255:bool)
            n5159 = local write "SEM Shutter"(w4257) -> ()
            n5160 = local write "SEM shutter failed active"(w4255) -> ()
          }
          event "Shtr Tune": Value Change {
            n5161 = event-data() -> ()  [unwired: 2 out]
            n5162 = flat-sequence {
              frame #0 {
                n5163 = local read "Hardware Configuration"() -> (w4265:T25)
                n5164 = Unbundle By Name(w4265) -> ("Shutter Drive"=w4264:tag, "Configuration file"=w4263:path)
                n5165 = call "Shutter Tuning Interface.vi"("Shutter Drive"=w4264, "Damping"="Damping", "configuration file path"=w4263) -> ("SEM shutter status"=w4266:string, "Damping out"=w4262:bool)  [unwired: 7 in]
                n5166 = local write "Damping"(w4262) -> ()
                n5167 = local write "SEM shutter status"(w4266) -> ()
              }
              frame #1 {
                n5168 = local write "Shtr Tune"(FALSE ("Shtr Tune")) -> ()
              }
            }
          }
          event "FIB Profile": Value Change {
            n5169 = event-data() -> ("NewVal"=w4269:bool)  [unwired: 1 out]
            n5170 = case shown="True" w4269 {
              frame False {
              }
              frame True {
                n5171 = Two Button Dialog(message="Characterize FIB Beam Profile?") -> (T button?=w4270:bool)  [unwired: 2 in]
                n5172 = case shown="True" w4270 {
                  frame False {
                    n5173 = local write "FIB Profile"(FALSE ("FIB Profile")) -> ()
                  }
                  frame True {
                    n5174 = stacked-sequence {
                      frame #0 {
                        n5175 = local read "Enable logging"() -> (→"Logging status before profiling":bool)
                      }
                      frame #1 {
                        n5176 = local write "Enable logging"(FALSE ("Enable logging")) -> ()
                        n5177 = Wait (ms)(milliseconds to wait=u32 200) -> ()  [unwired: 1 out]
                        n5178 = local write "Image Tabs"(T37."Logging: Realtime Graphs" ("Image Tabs")) -> ()
                      }
                      frame #2 {
                        n5179 = local read "Machine Type"() -> (w4277:u8)
                        n5180 = case shown="2" w4277 {
                          frame 0, Default {
                            n5181 = local read "HV Data Output"() -> (w4283:T18)
                            n5182 = local read "FIB HW Config"() -> (w4291:T23)
                            n5183 = local read "FIB Options"() -> (w4289:T33)
                            n5184 = local read "Milling para"() -> (w4290:T35)
                            n5185 = local read "FIB Scan Parameters"() -> (w4293:T32)
                            n5186 = local read "Parameter Names"() -> (w4286:string[])
                            n5187 = Bundle By Name(cluster=w4293, "Frame line rampdown ratio"=0.0, "Oversampling"=u16 5) -> (w4288:T32)
                            n5188 = local read "Active logging channels"() -> (w4287:string)
                            n5189 = local read "Api"() -> (w4282:refnum<k7>)
                            n5190 = call "FIB profile.vi"("ActiveX Container"=w4282, "HV Data Output"=w4283, "Parameter Names"=w4286, "Active logging channels"=w4287, "Scan Para"=w4288, "Milling para"=w4290, "Options"=w4289, "HW Config"=w4291) -> ("Measurements"=w4285:dbl[][])  [unwired: 1 in, 2 out]
                            n5191 = local write "Measurements"(w4285) -> ()
                          }
                          frame 2 {
                            n5192 = local read "FIB HW Config"() -> (w4303:T23)
                            n5193 = local read "FIB Options"() -> (w4301:T33)
                            n5194 = local read "Milling para"() -> (w4302:T35)
                            n5195 = local read "FIB Scan Parameters"() -> (w4305:T32)
                            n5196 = local read "Parameter Names"() -> (w4298:string[])
                            n5197 = local read "Capella HV Data Output"() -> (w4295:T17)
                            n5198 = Bundle By Name(cluster=w4305, "Frame line rampdown ratio"=0.0, "Oversampling"=u16 5) -> (w4300:T32)
                            n5199 = local read "Active logging channels"() -> (w4299:string)
                            n5200 = local read "Api"() -> (w4294:refnum<k7>)
                            n5201 = call "FIB profile.vi"("ActiveX Container"=w4294, "Capella HV Data Output"=w4295, "Parameter Names"=w4298, "Active logging channels"=w4299, "Scan Para"=w4300, "Milling para"=w4302, "Options"=w4301, "HW Config"=w4303) -> ("Measurements"=w4297:dbl[][])  [unwired: 1 in, 2 out]
                            n5202 = local write "Measurements"(w4297) -> ()
                          }
                        }
